vi "String to locale number.vi"(10 "numberString":string) -> (2 "locale string":string, 3 "locale number":dbl, 5 "locale decimal separator":string, 7 "non-locale decimal separator":string)   [LabVIEW 2018]
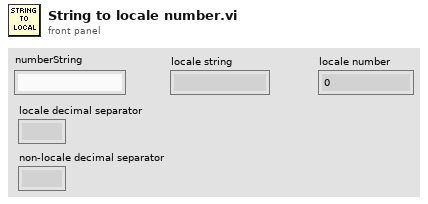
[diagram p1: front panel]
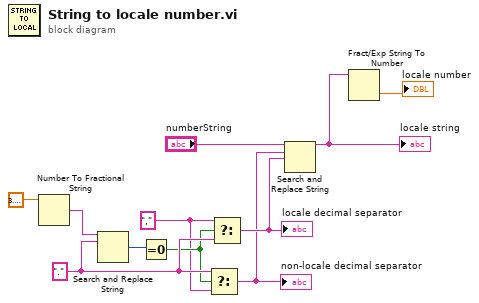
[diagram p0: block diagram]
diagram:
  w4 = "," ("t")
  w6 = "." ("regular expression")
  n1 = Number To Fractional String(number=3.141592653589793) -> (F-format string=w10:string)  [unwired: 3 in]
  n2 = Search and Replace String(input string=w10, search string=w6) -> (number of replacements=w9:i32)  [unwired: 6 in, 3 out]
  n3 = Equal To 0?(x=w9) -> (x = 0?=w5:bool)
  n4 = Select(t=w6, s=w5, f=w4) -> (s? t:f=w3:string)
  "non-locale decimal separator" <- w3
  n5 = Select(t=w4, s=w5, f=w6) -> (s? t:f=w7:string)
  "locale decimal separator" <- w7
  n6 = Search and Replace String(input string="numberString", search string=w3, replace string=w7) -> (result string=w2:string)  [unwired: 5 in, 3 out]
  "locale string" <- w2
  n7 = Fract/Exp String To Number(string=w2) -> (number=→"locale number":dbl)  [unwired: 3 in, 1 out]
